vi "spec_set_mass.vi"(8 "error in (no error)":errorcluster, 10 "mass":dbl, 11 "Qtegra in":refnum<class "Qtegra.lvclass">) -> (0 "error out":errorcluster, 2 "data out":string, 3 "Qtegra out":refnum<class "Qtegra.lvclass">)   [LabVIEW 2018, in "Qtegra.lvclass"]
uses:
  Qtegra.lvclass
  \\Mac\Home/my data/privat/Software/LabView/MSControlSuite_Code/MSControl/Classes/Instrument/instrument.lvclass
  global variables.vi
  instrument.lvclass
  StatusLog/StatusLog.lvclass
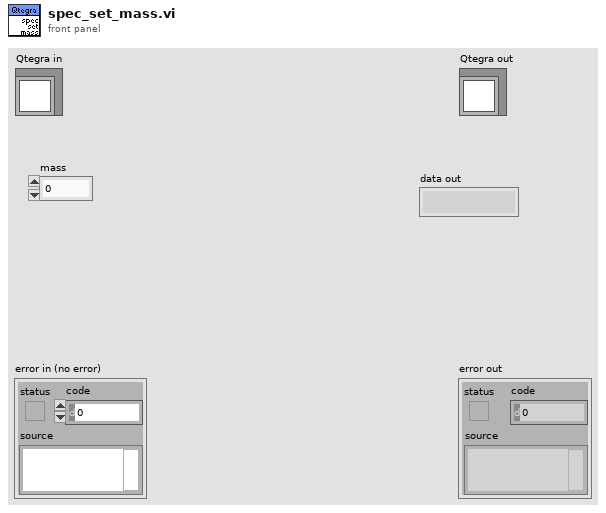
[diagram p1: front panel]
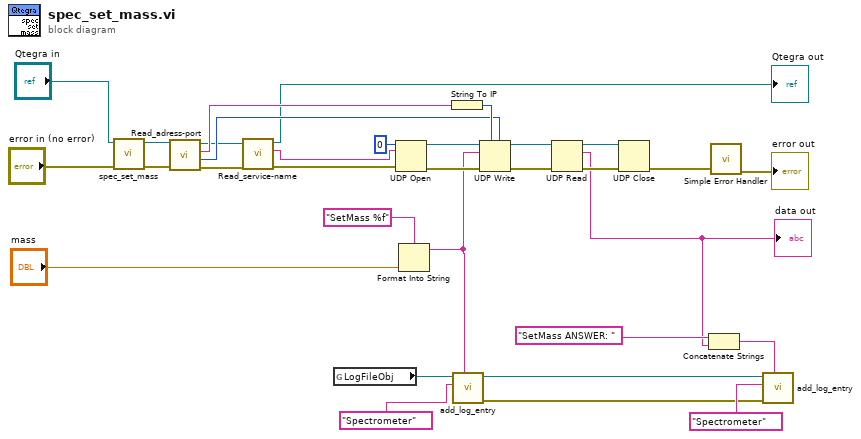
[diagram p0: block diagram]
diagram:
  n1 = call-parent "spec_set_mass.vi"("error in (no error)"="error in (no error)", "instrument in"="Qtegra in") -> ("error out"=w17:errorcluster, "instrument out"=w18:refnum<class "Qtegra.lvclass">)  [unwired: 7 in, 1 out]
  n2 = call "Read_adress-port.vi"("error in (no error)"=w17, "instrument in"=w18) -> ("error out"=w22:errorcluster, "port number"=w23:i32, "adress"=w30:string, "instrument out"=w21:refnum<class "Qtegra.lvclass">)  [unwired: 6 in]
  n3 = call-dynamic "Read_service-name.vi"("error in (no error)"=w22, "instrument in"=w21) -> ("error out"=w20:errorcluster, "service name"=w19:string, "instrument out"=→"Qtegra out":refnum<class "Qtegra.lvclass">)  [unwired: 7 in]
  n4 = global read "global variables.vi" "LogFileObj"() -> (w7:refnum<class "StatusLog.lvclass">)
  n5 = UDP Open(8:w20, 10:w19, 11:u16 0 ("port")) -> (port=w26:refnum<k16>, 0:w27:errorcluster)  [unwired: 2 in, 1 out]
  n6 = Format Into String(format string="SetMass %f", "mass") -> (resulting string=w2:string)  [unwired: 2 in, 1 out]
  n7 = String To IP(1:w30) -> (0:w29:u32)
  n8 = call-dynamic "add_log_entry.vi"("new entry"=w2, "log identifiers"="Spectrometer", "StatusLog in"=w7) -> ("error out"=w3:errorcluster, "StatusLog out"=w6:refnum<class "StatusLog.lvclass">)  [unwired: 5 in]
  n9 = UDP Write(address=w29, port or service name=w23, connection ID=w26, data in=w2, 8:w27) -> (error out=w24:errorcluster, 3:w25:refnum<k16>)  [unwired: 1 in]
  n10 = UDP Read(connection ID=w25, 8:w24) -> (data out=w1:string, error out=w11:errorcluster, 3:w12:refnum<k16>)  [unwired: 2 in, 2 out]
  "data out" <- w1
  n11 = UDP Close(connection ID=w12, 8:w11) -> (error out=w10:errorcluster)  [unwired: 1 out]
  n12 = Concatenate Strings("SetMass ANSWER: ", w1) -> (w4:string)
  n13 = call <vilib>:"Simple Error Handler.vi"("error in (no error)"=w10) -> ("error out"=→"error out":errorcluster)  [unwired: 4 in, 4 out]
  n14 = call-dynamic "add_log_entry.vi"("new entry"=w4, "error in (no error)"=w3, "log identifiers"="Spectrometer", "StatusLog in"=w6) -> ()  [unwired: 4 in, 2 out]
